vi "GetTopLevelControlTerminalRefs.vi"(8 "error in (no error)":errorcluster, 11 "VI ref in":refnum<vi>) -> (0 "error out":errorcluster, 2 "Control terminals on top-level":refnum<vi>[](array[refnum]), 3 "VI ref out (dup)":refnum<vi>)   [LabVIEW 2017, in "ErrorStructureDrawer.lvlib"]
doc: "Get references to control terminals who are owned by the top level diagram of the specified VI"
uses:
  <vilib>/Utility/traverseref.llb/TRef TravTarget.ctl
  ErrorStructureDrawer.lvlib
  <vilib>/Utility/traverseref.llb/VI Scripting - Traverse.lvlib
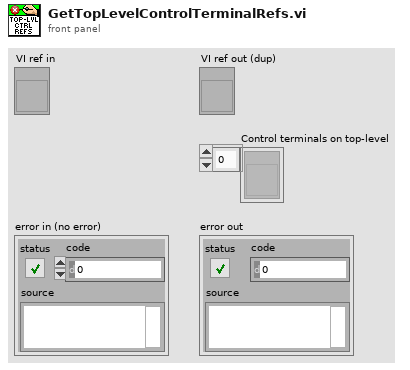
[diagram p1: front panel]
types:
  T1 = typedef "TRef TravTarget.ctl" = enum16{"FP", "BD", "Other"}
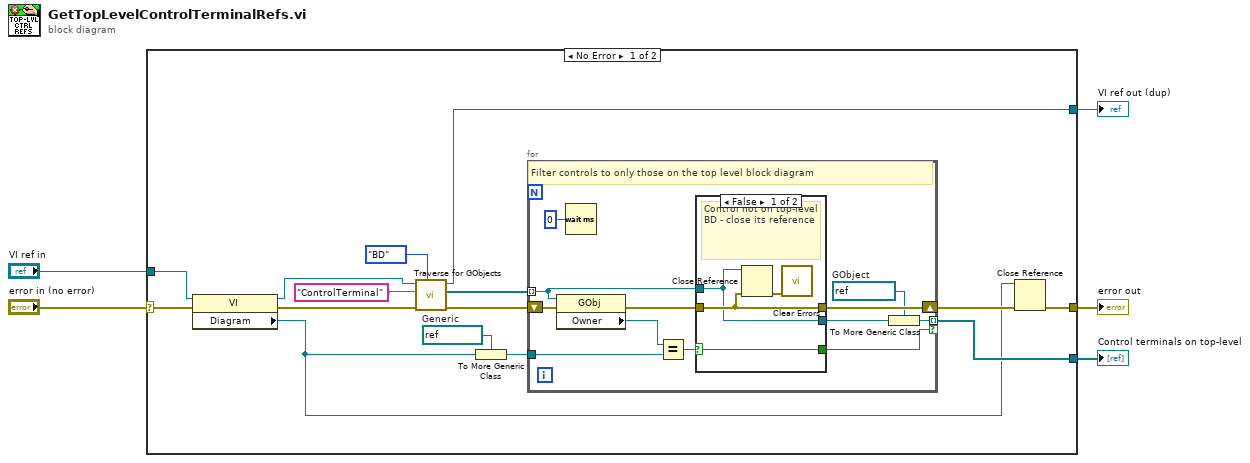
[diagram p0: block diagram]
diagram:
  n1 = case shown="No Error" "error in (no error)" {
    selector: "error in (no error)" -> [w6 w41]
    tunnel: [w20 w40] -> w5
    tunnel: [w19 _] -> w4
    tunnel: "VI ref in" -> [w10 w40]
    tunnel: [w8 w41] -> w2
    frame No Error {
      w15 = refnum<vi> refnum  # Generic
      n2 = property class="VI"(reference=w10, error in=w6) -> (reference out=w9:refnum<vi>, error out=w11:errorcluster, "Diagram"=w7:refnum<vi>)
      n3 = call <vilib>:"Traverse for GObjects.vi"("Traverse Target"=TRef_TravTarget."BD", "error in (no error)"=w11, "Class Name"="ControlTerminal", "VI Refnum"=w9) -> ("error out"=w14:errorcluster, "References"=w17:refnum<vi>[], "dup VI Refnum"=w20:refnum<vi>)  [unwired: 4 in, 1 out]
      n4 = To More Generic Class(target class=w15, reference=w7) -> (generic class reference=w16:refnum<vi>)
      n5 = for {
        tunnel: w17 -> [w28] mode=indexing
        shift-right: [w30] -> w18
        shift-left: w14 -> [w32]
        tunnel: w16 -> [w31]
        tunnel: [w22] -> w19 mode=indexing if=w29
        w24 = refnum<vi> refnum  # GObject
        # "Filter controls to only those on the top level block diagram"
        n6 = property class="GObj"(reference=w28, error in=w32) -> (error out=w27:errorcluster, "Owner"=w26:refnum<vi>)  [unwired: 1 out]
        n7 = Wait (ms)(milliseconds to wait=u32 0) -> ()  [unwired: 1 out]
        n8 = Equal?(x=w26, y=w31) -> (x = y?=w25:bool)
        n9 = case shown="False" w25 {
          selector: w25 -> [w34 w37]
          tunnel: w27 -> [w35 w39]
          tunnel: [w35 w39] -> w30
          tunnel: [w34 w37] -> w29
          tunnel: [w33 w38] -> w23
          tunnel: w28 -> [w33 w38]
          frame False {
            # "Control not on top-level BD - close its reference"
            n10 = Close Reference(reference=w33, error in (no error)=w35) -> (error out=w36:errorcluster)
            n11 = call <vilib>:"Clear Errors.vi"("error in (no error)"=w36) -> ()  [unwired: 5 in, 2 out]
          }
          frame True {
            # "Control is on top-level BD, do nothing here"
          }
        }
        n12 = To More Generic Class(target class=w24, reference=w23) -> (generic class reference=w22:refnum<vi>)
      }
      n13 = Close Reference(reference=w7, error in (no error)=w18) -> (error out=w8:errorcluster)
    }
    frame Error {
    }
  }
  "VI ref out (dup)" <- w5
  "Control terminals on top-level" <- w4
  "error out" <- w2
